vi "force_control_loop_3axis_indiv.vi"(0 "Force In":dbl[](array[numeric]), 5 "Goal Position IN":dbl[][](array[numeric]), 7 "Force Stimulus":dbl[](array[numeric]), 9 "Control Axis":enum16{"x axis", "y axis", "z axis"}(ring), 11 "Force Control Type":T1(ring), 12 "Ki Degradation":dbl) -> (6 "Force Position Out":dbl[](array[numeric]), 15 "Last Error":dbl[](array[numeric]))   [LabVIEW 2014]
uses:
  <vilib>/Analysis/Matrix/Datatypes/RealMatrix.ctl
  <vilib>/Analysis/baseanly.llb/Real A x B.vi
  force_control_globals.vi
  <vilib>/Analysis/Matrix/Numeric/Conversions/Matrix To Array - RM.vi
  <vilib>/Analysis/NI_AALBase.lvlib
  <vilib>/Analysis/Matrix/NI_Matrix.lvlib
panel:
  out "Goal Position HOLD":dbl[][](array[numeric])
  out "Last dForce":dbl[](array[numeric])
  out "Inject Stimulus":bool
  out "Last Force":dbl[](array[numeric])
  in  "Accel Transform":T2
  out "Last Ki":dbl[](array[numeric])
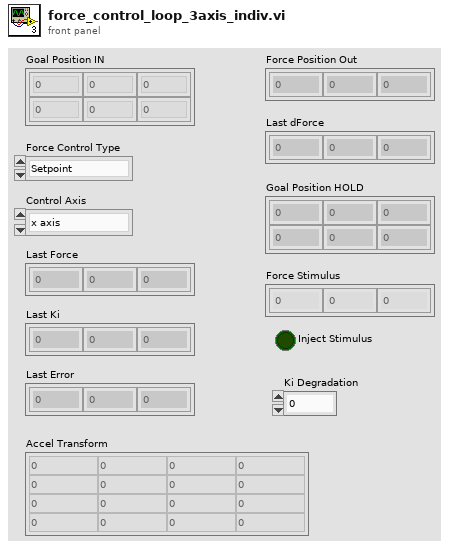
[diagram p1: front panel]
types:
  T1 = enum16{"Setpoint", "One Way Threshold", "Two Way Threshold"}
  T2 = typedef "NI_Matrix.lvlib/RealMatrix.ctl" = dbl[][]
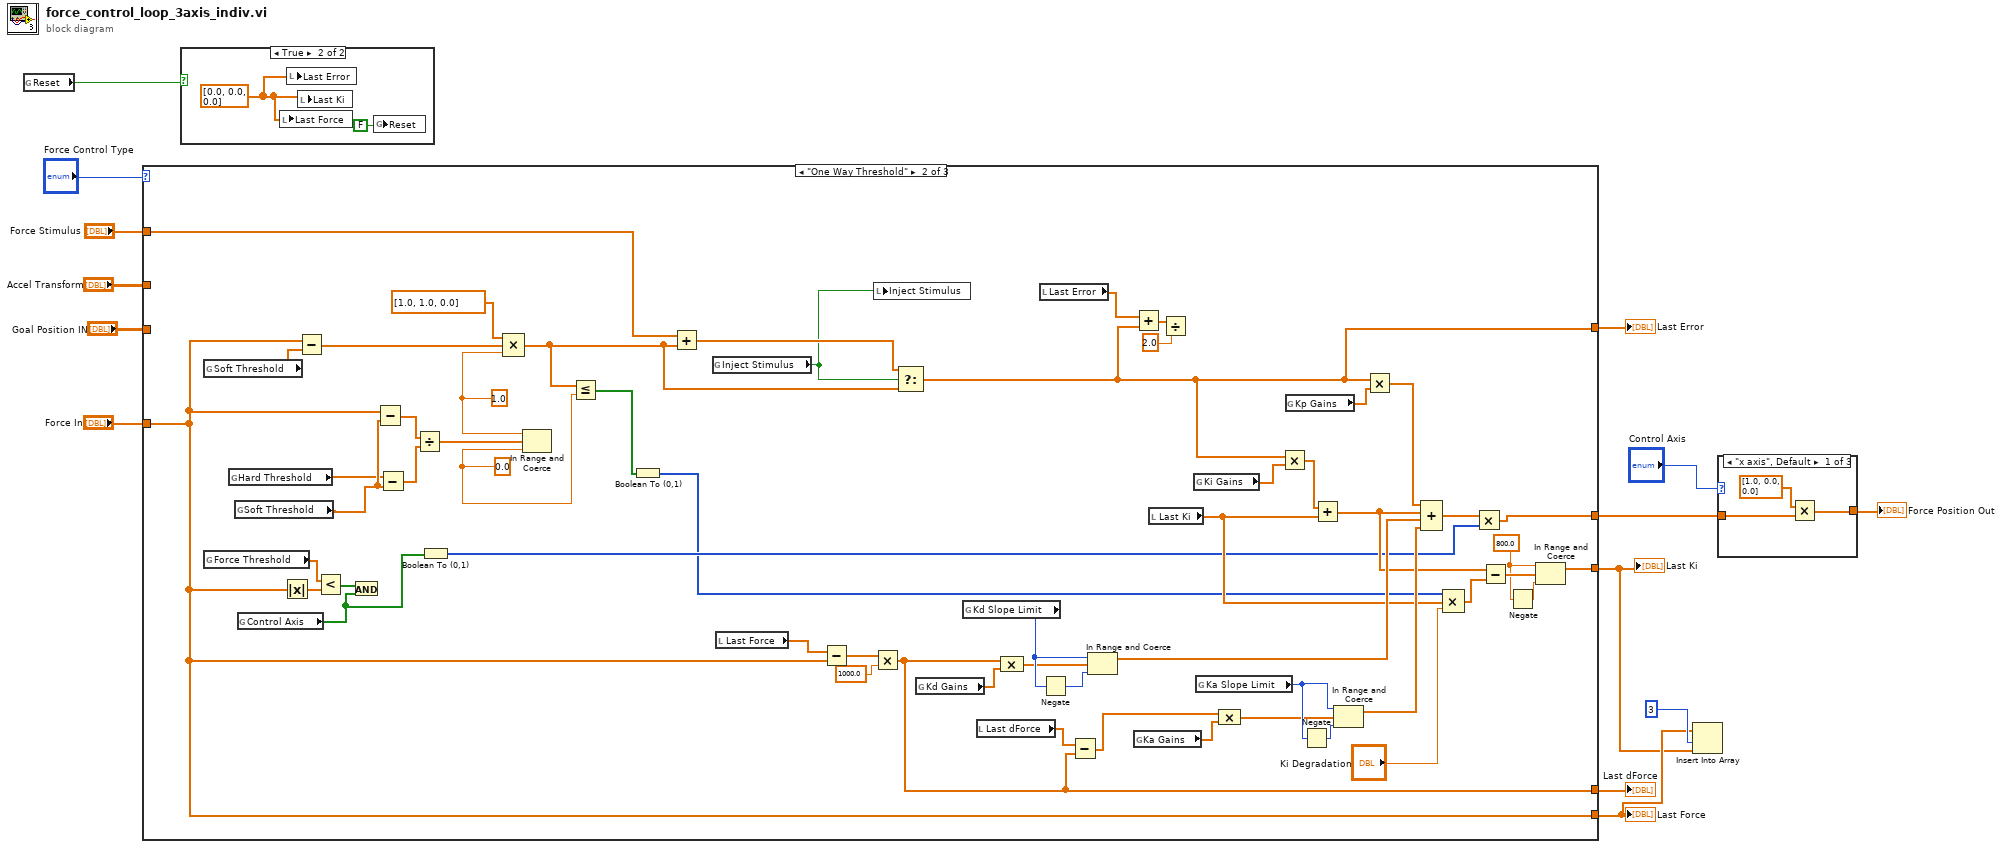
[diagram p0: block diagram]
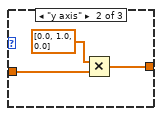
[diagram p2: hidden frame]
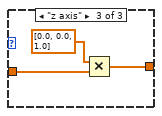
[diagram p3: hidden frame]
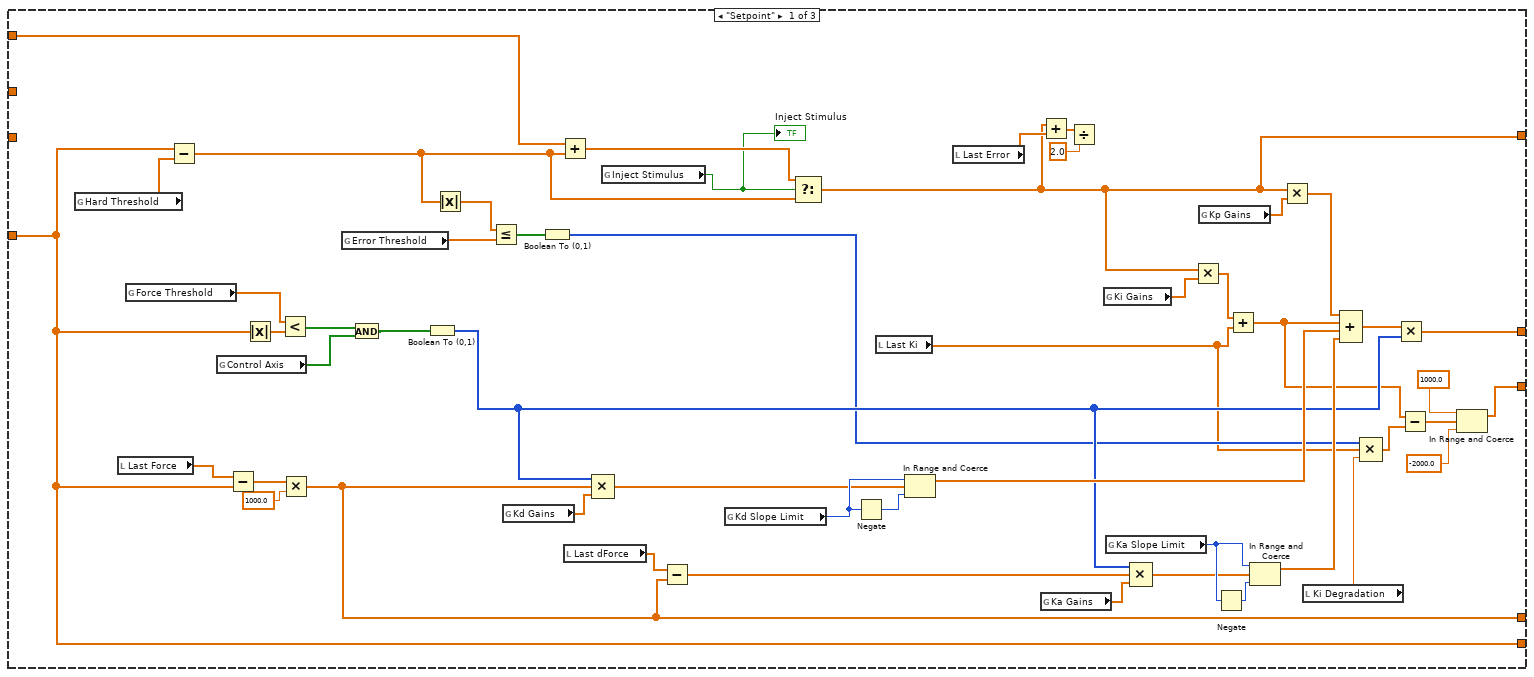
[diagram p5: hidden frame]
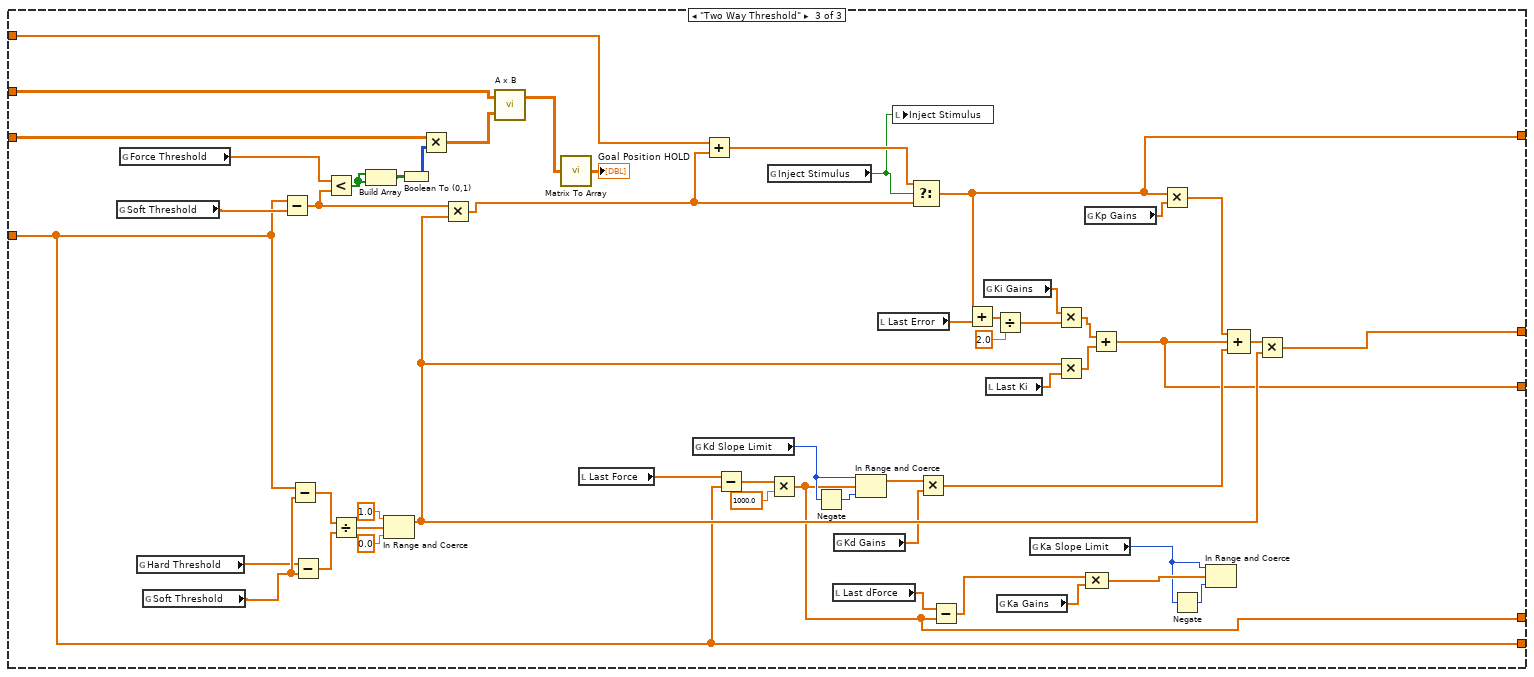
[diagram p6: hidden frame]
diagram:
  n1 = global read "force_control_globals.vi" "Reset"() -> (w9:bool)
  n2 = case shown="\"One Way Threshold\"" "Force Control Type" {
    tunnel: "Force In" -> [w47 w88 w124]
    tunnel: [w17 w70 w121] -> w1
    tunnel: [w41 w83 w159] -> w3
    tunnel: [w43 w71 w157] -> w2
    tunnel: "Accel Transform" -> [_ _ w144]
    tunnel: "Force Stimulus" -> [w53 w110 w132]
    tunnel: [w47 w88 w124] -> w4
    tunnel: "Goal Position IN" -> [_ _ w130]
    tunnel: [w38 w99 w123] -> w10
    frame "Setpoint" {
      n3 = global read "force_control_globals.vi" "Hard Threshold"() -> (w51:sgl[])
      n4 = local read "Last Force"() -> (w59:dbl[])
      n5 = global read "force_control_globals.vi" "Force Threshold"() -> (w32:sgl[])
      n6 = Subtract(x=w47, y=w51) -> (x-y=w27:dbl[])
      n7 = global read "force_control_globals.vi" "Control Axis"() -> (w29:bool[])
      n8 = Subtract(x=w59, y=w47) -> (x-y=w61:dbl[])
      n9 = Absolute Value(x=w47) -> (abs(x)=w64:dbl[])
      n10 = Less?(x=w32, y=w64) -> (x < y?=w30:bool[])
      n11 = Multiply(x=w61, y=1000.0) -> (x*y=w38:dbl[])
      n12 = global read "force_control_globals.vi" "Error Threshold"() -> (w25:sgl[])
      n13 = And(x=w30, y=w29) -> (x .and. y?=w31:bool[])
      n14 = Boolean To (0,1)(Boolean=w31) -> (0, 1=w28:i16[])
      n15 = Absolute Value(x=w27) -> (abs(x)=w26:dbl[])
      n16 = Less Or Equal?(x=w26, y=w25) -> (x <= y?=w24:bool[])
      n17 = global read "force_control_globals.vi" "Kd Gains"() -> (w50:sgl[])
      n18 = Boolean To (0,1)(Boolean=w24) -> (0, 1=w20:i16[])
      n19 = Add(x=w53, y=w27) -> (x+y=w63:dbl[])
      n20 = local read "Last dForce"() -> (w39:dbl[])
      n21 = Compound Arithmetic op=MULTIPLY(w28, w38, w50) -> (w45:dbl[])
      n22 = global read "force_control_globals.vi" "Inject Stimulus"() -> (w49:bool)
      "Inject Stimulus" <- w49
      n23 = Subtract(x=w39, y=w38) -> (x-y=w37:dbl[])
      n24 = global read "force_control_globals.vi" "Kd Slope Limit"() -> (w46:i32)
      n25 = Select(t=w63, s=w49, f=w27) -> (s? t:f=w41:dbl[])
      n26 = Negate(x=w46) -> (-x=w58:i32)
      n27 = local read "Last Ki"() -> (w19:dbl[])
      n28 = In Range and Coerce(upper limit=w46, x=w45, lower limit=w58) -> (coerced(x)=w44:dbl[])  [unwired: 1 out]
      n29 = local read "Last Error"() -> (w55:dbl[])
      n30 = Add(x=w41, y=w55) -> (x+y=w56:dbl[])
      n31 = global read "force_control_globals.vi" "Ka Gains"() -> (w40:sgl[])
      n32 = Divide(x=w56, y=2.0) -> ()  [unwired: 1 out]
      n33 = global read "force_control_globals.vi" "Ki Gains"() -> (w48:sgl[])
      n34 = global read "force_control_globals.vi" "Ka Slope Limit"() -> (w35:i32)
      n35 = Compound Arithmetic op=MULTIPLY(w28, w37, w40) -> (w34:dbl[])
      n36 = Multiply(x=w41, y=w48) -> (x*y=w54:dbl[])
      n37 = global read "force_control_globals.vi" "Kp Gains"() -> (w52:sgl[])
      n38 = Negate(x=w35) -> (-x=w36:i32)
      n39 = Add(x=w54, y=w19) -> (x+y=w18:dbl[])
      n40 = In Range and Coerce(upper limit=w35, x=w34, lower limit=w36) -> (coerced(x)=w33:dbl[])  [unwired: 1 out]
      n41 = Multiply(x=w41, y=w52) -> (x*y=w62:dbl[])
      n42 = local read "Ki Degradation"() -> (w16:dbl)
      n43 = Compound Arithmetic op=ADD(w62, w18, w44, w33) -> (w42:dbl[])
      n44 = Compound Arithmetic op=MULTIPLY(w20, w19, w16) -> (w23:dbl[])
      n45 = Multiply(x=w42, y=w28) -> (x*y=w43:dbl[])
      n46 = Subtract(x=w18, y=w23) -> (x-y=w22:dbl[])
      n47 = In Range and Coerce(upper limit=1000.0, x=w22, lower limit=-2000.0) -> (coerced(x)=w17:dbl[])  [unwired: 1 out]
    }
    frame "One Way Threshold" {
      w67 = 800.0
      w84 = 1.0 ("upper limit")
      w74 = 0.0 ("lower limit")
      n48 = global read "force_control_globals.vi" "Soft Threshold"() -> (w108:sgl[])
      n49 = global read "force_control_globals.vi" "Force Threshold"() -> (w93:sgl[])
      n50 = global read "force_control_globals.vi" "Hard Threshold"() -> (w90:sgl[])
      n51 = global read "force_control_globals.vi" "Soft Threshold"() -> (w91:sgl[])
      n52 = global read "force_control_globals.vi" "Control Axis"() -> (w75:bool[])
      n53 = Absolute Value(x=w88) -> (abs(x)=w120:dbl[])
      n54 = Subtract(x=w88, y=w108) -> (x-y=w87:dbl[])
      n55 = Less?(x=w93, y=w120) -> (x < y?=w82:bool[])
      n56 = And(x=w82, y=w75) -> ()  [unwired: 1 out]
      n57 = Subtract(x=w88, y=w91) -> (x-y=w89:dbl[])
      n58 = Subtract(x=w90, y=w91) -> (x-y=w76:sgl[])
      n59 = Divide(x=w89, y=w76) -> (x/y=w92:dbl[])
      n60 = Boolean To (0,1)(Boolean=w75) -> (0, 1=w73:i16[])
      n61 = Compound Arithmetic op=MULTIPLY(dbl[] [1.0, 1.0, 0.0], w87, w84) -> (w78:dbl[])
      n62 = In Range and Coerce(upper limit=w84, x=w92, lower limit=w74) -> ()  [unwired: 2 out]
      n63 = Less Or Equal?(x=w78, y=w74) -> (x <= y?=w77:bool[])
      n64 = Boolean To (0,1)(Boolean=w77) -> (0, 1=w72:i16[])
      n65 = Add(x=w110, y=w78) -> (x+y=w119:dbl[])
      n66 = global read "force_control_globals.vi" "Inject Stimulus"() -> (w86:bool)
      n67 = local read "Last Force"() -> (w115:dbl[])
      n68 = Subtract(x=w115, y=w88) -> (x-y=w117:dbl[])
      n69 = Multiply(x=w117, y=1000.0) -> (x*y=w99:dbl[])
      n70 = local write "Inject Stimulus"(w86) -> ()
      n71 = Select(t=w119, s=w86, f=w78) -> (s? t:f=w83:dbl[])
      n72 = global read "force_control_globals.vi" "Kd Gains"() -> (w107:sgl[])
      n73 = global read "force_control_globals.vi" "Kd Slope Limit"() -> (w105:i32)
      n74 = local read "Last dForce"() -> (w100:dbl[])
      n75 = Compound Arithmetic op=MULTIPLY(w99, w107) -> (w104:dbl[])
      n76 = local read "Last Error"() -> (w85:dbl[])
      n77 = Negate(x=w105) -> (-x=w114:i32)
      n78 = Subtract(x=w100, y=w99) -> (x-y=w98:dbl[])
      n79 = In Range and Coerce(upper limit=w105, x=w104, lower limit=w114) -> (coerced(x)=w103:dbl[])  [unwired: 1 out]
      n80 = Add(x=w85, y=w83) -> (x+y=w112:dbl[])
      n81 = global read "force_control_globals.vi" "Ka Gains"() -> (w101:sgl[])
      n82 = local read "Last Ki"() -> (w80:dbl[])
      n83 = Divide(x=w112, y=2.0) -> ()  [unwired: 1 out]
      n84 = global read "force_control_globals.vi" "Ki Gains"() -> (w106:sgl[])
      n85 = global read "force_control_globals.vi" "Ka Slope Limit"() -> (w96:i32)
      n86 = Compound Arithmetic op=MULTIPLY(w98, w101) -> (w95:dbl[])
      n87 = Multiply(x=w83, y=w106) -> (x*y=w111:dbl[])
      n88 = global read "force_control_globals.vi" "Kp Gains"() -> (w109:sgl[])
      n89 = Negate(x=w96) -> (-x=w97:i32)
      n90 = Add(x=w111, y=w80) -> (x+y=w81:dbl[])
      n91 = In Range and Coerce(upper limit=w96, x=w95, lower limit=w97) -> (coerced(x)=w94:dbl[])  [unwired: 1 out]
      n92 = Multiply(x=w83, y=w109) -> (x*y=w118:dbl[])
      n93 = Compound Arithmetic op=ADD(w118, w81, w103, w94) -> (w102:dbl[])
      n94 = Compound Arithmetic op=MULTIPLY(w72, w80, "Ki Degradation") -> (w79:dbl[])
      n95 = Multiply(x=w102, y=w73) -> (x*y=w71:dbl[])
      n96 = Subtract(x=w81, y=w79) -> (x-y=w69:dbl[])
      n97 = Negate(x=w67) -> (-x=w68:dbl)
      n98 = In Range and Coerce(upper limit=w67, x=w69, lower limit=w68) -> (coerced(x)=w70:dbl[])  [unwired: 1 out]
    }
    frame "Two Way Threshold" {
      n99 = global read "force_control_globals.vi" "Soft Threshold"() -> (w134:sgl[])
      n100 = global read "force_control_globals.vi" "Force Threshold"() -> (w133:sgl[])
      n101 = global read "force_control_globals.vi" "Hard Threshold"() -> (w135:sgl[])
      n102 = global read "force_control_globals.vi" "Soft Threshold"() -> (w136:sgl[])
      n103 = Subtract(x=w124, y=w134) -> (x-y=w148:dbl[])
      n104 = Subtract(x=w124, y=w136) -> (x-y=w153:dbl[])
      n105 = Subtract(x=w135, y=w136) -> (x-y=w152:sgl[])
      n106 = Less?(x=w133, y=w148) -> (x < y?=w147:bool[])
      n107 = Divide(x=w153, y=w152) -> (x/y=w151:dbl[])
      n108 = Build Array(w147, w147) -> (w145:bool[][])
      n109 = In Range and Coerce(upper limit=1.0, x=w151, lower limit=0.0) -> (coerced(x)=w149:dbl[])  [unwired: 1 out]
      n110 = Boolean To (0,1)(Boolean=w145) -> (0, 1=w146:i16[][])
      n111 = Multiply(x=w130, y=w146) -> (x*y=w143:dbl[][])
      n112 = Multiply(x=w148, y=w149) -> (x*y=w150:dbl[])
      n113 = call-poly <vilib>:"A x B.vi"("B"=w143, "A"=w144) -> ("A x B"=w141:T2)  [unwired: 1 out]
      n114 = call-poly <vilib>:"Matrix To Array.vi"("Real Matrix"=w141) -> ("Real 2D Array"=→"Goal Position HOLD":dbl[][])
      n115 = local read "Last Force"() -> (w168:dbl[])
      n116 = global read "force_control_globals.vi" "Kd Slope Limit"() -> (w137:i32)
      n117 = Add(x=w132, y=w150) -> (x+y=w173:dbl[])
      n118 = Subtract(x=w168, y=w124) -> (x-y=w170:dbl[])
      n119 = global read "force_control_globals.vi" "Inject Stimulus"() -> (w131:bool)
      n120 = Multiply(x=w170, y=1000.0) -> (x*y=w123:dbl[])
      n121 = Negate(x=w137) -> (-x=w167:i32)
      n122 = local read "Last dForce"() -> (w128:dbl[])
      n123 = global read "force_control_globals.vi" "Kd Gains"() -> (w138:sgl[])
      n124 = In Range and Coerce(upper limit=w137, x=w123, lower limit=w167) -> (coerced(x)=w166:dbl[])  [unwired: 1 out]
      n125 = local read "Last Error"() -> (w161:dbl[])
      n126 = local write "Inject Stimulus"(w131) -> ()
      n127 = Select(t=w173, s=w131, f=w150) -> (s? t:f=w159:dbl[])
      n128 = Multiply(x=w166, y=w138) -> (x*y=w171:dbl[])
      n129 = Subtract(x=w128, y=w123) -> (x-y=w127:dbl[])
      n130 = Add(x=w159, y=w161) -> (x+y=w162:dbl[])
      n131 = global read "force_control_globals.vi" "Ki Gains"() -> (w139:sgl[])
      n132 = local read "Last Ki"() -> (w164:dbl[])
      n133 = Divide(x=w162, y=2.0) -> (x/y=w160:dbl[])
      n134 = global read "force_control_globals.vi" "Ka Gains"() -> (w129:sgl[])
      n135 = global read "force_control_globals.vi" "Ka Slope Limit"() -> (w122:i32)
      n136 = Multiply(x=w139, y=w160) -> (x*y=w156:dbl[])
      n137 = Multiply(x=w149, y=w164) -> (x*y=w165:dbl[])
      n138 = global read "force_control_globals.vi" "Kp Gains"() -> (w140:sgl[])
      n139 = Compound Arithmetic op=MULTIPLY(w127, w129) -> (w125:dbl[])
      n140 = Add(x=w156, y=w165) -> (x+y=w121:dbl[])
      n141 = Multiply(x=w159, y=w140) -> (x*y=w172:dbl[])
      n142 = Negate(x=w122) -> (-x=w126:i32)
      n143 = In Range and Coerce(upper limit=w122, x=w125, lower limit=w126) -> ()  [unwired: 2 out]
      n144 = Compound Arithmetic op=ADD(w172, w121, w171) -> (w158:dbl[])
      n145 = Multiply(x=w158, y=w149) -> (x*y=w157:dbl[])
    }
  }
  "Last Error" <- w3
  "Last Ki" <- w1
  "Last Force" <- w4
  "Last dForce" <- w10
  n146 = case shown="True" w9 {
    frame False {
    }
    frame True {
      w175 = dbl[] [0.0, 0.0, 0.0]
      n147 = local write "Last Force"(w175) -> ()
      n148 = local write "Last Error"(w175) -> ()
      n149 = local write "Last Ki"(w175) -> ()
      n150 = global write "force_control_globals.vi" "Reset"(FALSE) -> ()
    }
  }
  n151 = Insert Into Array(array=w4, index=3, new element=w1) -> ()  [unwired: 1 out]
  n152 = case shown="\"x axis\", Default" "Control Axis" {
    tunnel: w2 -> [w177 w180 w183]
    tunnel: [w176 w179 w182] -> w6
    frame "x axis", Default {
      n153 = Multiply(x=dbl[] [1.0, 0.0, 0.0], y=w177) -> (x*y=w176:dbl[])
    }
    frame "y axis" {
      n154 = Multiply(x=dbl[] [0.0, 1.0, 0.0], y=w180) -> (x*y=w179:dbl[])
    }
    frame "z axis" {
      n155 = Multiply(x=dbl[] [0.0, 0.0, 1.0], y=w183) -> (x*y=w182:dbl[])
    }
  }
  "Force Position Out" <- w6
